vi "InitSensors.vi"   [LabVIEW 2019]
uses:
  <vilib>/Rock Robotics/SystemInterfaces/AI/FPGA_AIChannel.ctl
  <vilib>/Rock Robotics/WPI/ThirdParty/Phoenix-LabVIEW/Pigeon IMU/CTRE_PigeonIMU_TareType.ctl
  <vilib>/Rock Robotics/SystemInterfaces/DIO/FPGA_DIOChannel.ctl
  refnums.vi
  <vilib>/Rock Robotics/WPI/Counter/WPI_CounterDigitalInputToDigitalSource.vi
  <vilib>/Rock Robotics/WPI/Counter/WPI_CounterOpen UpDown Mode.vi
  <vilib>/Rock Robotics/WPI/Switch/WPI_SwitchOpenLimit.vi
  <vilib>/Rock Robotics/WPI/ThirdParty/Phoenix-LabVIEW/Pigeon IMU/CTRE_PigeonIMU_Open_TalonSRX.vi
types:
  T1 = typedef "FPGA_DIOChannel.ctl" = enum8{"DIO 0", "DIO 1", "DIO 2", "DIO 3", "DIO 4", "DIO 5", "DIO 6", "DIO 7", "DIO 8", "DIO 9", "DIO MXP 0", "DIO MXP 1", "DIO MXP 2", "DIO MXP 3", "DIO MXP 4", "DIO MXP 5", "DIO MXP 6", "DIO MXP 7", "DIO MXP 8", "DIO MXP 9", "DIO MXP 10", "DIO MXP 11", "DIO MXP 12", "DIO MXP 13", "DIO MXP 14", "DIO MXP 15", "SPI Port CS1", "SPI Port CS2", "SPI Port CS3", "SPI Port MISO", "SPI Port MOSI", "Invalid"}
  T2 = enum16{"Rising Edge", "Falling Edge", "Raising & Falling Edge", "Disabled"}
  T3 = typedef "FPGA_AIChannel.ctl" = enum8{"AI 0", "AI 1", "AI 2", "AI 3", "AI MXP 0", "AI MXP 1", "AI MXP 2", "AI MXP 3", "Invalid"}
  T4 = typedef "CTRE_PigeonIMU_TareType.ctl" = u8
  T5 = typedef "WPI_MotorControlDeviceRef.ctl" = cluster{"DeviceStatus":errorcluster, "Type":T6, "PWM":cluster{"PWM Channel":T7, "DeadBand":T8}, "CAN":cluster{"Device Number":u8, "SetOutput VI Ref":variant, "GetOutput VI Ref":variant, "Enable VI Ref":variant, "Disable VI Ref":variant, "Data":variant}, "Invert":bool, "DIO PWM":cluster{"PWM \"Enable\" Channel":T7, "DIOChannel":T1, "PWM Rate":dbl}}
  T6 = typedef "WPI_MotorControlType.ctl" = enum16{"PWM", "CAN", "DIO PWM"}
  T7 = typedef "FPGA_DIOPWMChannel.ctl" = enum8{"PWM 0", "PWM 1", "PWM 2", "PWM 3", "PWM 4", "PWM 5", "PWM 6", "PWM 7", "PWM 8", "PWM 9", "PWM MXP 0", "PWM MXP 1", "PWM MXP 2", "PWM MXP 3", "PWM MXP 4", "PWM MXP 5", "PWM MXP 6", "PWM MXP 7", "PWM MXP 8", "PWM MXP 9", "Invalid"}
  T8 = typedef "WPI_PWMDeadband.ctl" = cluster{"Name":string, "maxPositivePwm":i32, "minPositivePwm":i32, "centerPwm":i32, "maxNegativePwm":i32, "minNegativePwm":i32, "angularRange":u16}
  T9 = typedef "WPI_DigitalInputDevRef.ctl" = cluster{"DevStatus":errorcluster, "DIO Channel":T1}
  T10 = typedef "FPGA_CounterEncoderSourceConvertionLVSourceType.ctl" = cluster{"DevStatus":errorcluster, "AnalogTriggerMode?":bool, "DigitalMode":cluster{"DIO Channel":T11}, "AnalogTriggerMode":cluster{"AnalogTriggerIndex":T12, "OutputType":T13}}
  T11 = typedef "FPGA_DIODigitalSourceChannel.ctl" = enum8{"DIO 0", "DIO 1", "DIO 2", "DIO 3", "DIO 4", "DIO 5", "DIO 6", "DIO 7", "DIO 8", "DIO 9", "DIO MXP 0", "DIO MXP 1", "DIO MXP 2", "DIO MXP 3", "DIO MXP 4", "DIO MXP 5", "DIO MXP 6", "DIO MXP 7", "DIO MXP 8", "DIO MXP 9", "DIO MXP 10", "DIO MXP 11", "DIO MXP 12", "DIO MXP 13", "DIO MXP 14", "DIO MXP 15", "SPI Port CS1", "SPI Port CS2", "SPI Port CS3", "SPI Port MISO", "SPI Port MOSI", "Disabled"}
  T12 = typedef "FPGA_AnalogTriggerIndex.ctl" = enum8{"Trig 0", "Trig 1", "Trig 2", "Trig 3", "Trig 4", "Trig 5", "Trig 6", "Trig 7", "Invalid"}
  T13 = typedef "FPGA_AnalogTriggerOutType.ctl" = enum16{"InWindow", "TriggerState", "Rising", "Falling"}
  T14 = typedef "WPI_SwitchDevRef.ctl" = cluster{"DevStatus":errorcluster, "DIO Channel":T1, "CntIndex":T15, "Normally Closed":bool}
  T15 = typedef "FPGA_CounterCtrSystemIndex.ctl" = enum8{"Ctr 0", "Ctr 1", "Ctr 2", "Ctr 3", "Ctr 4", "Ctr 5", "Ctr 6", "Ctr 7", "Invalid"}
  T16 = typedef "WPI_PotentiometerDevRef.ctl" = cluster{"DevStatus":errorcluster, "Analog Channel":T3, "Invert Output":bool}
  T17 = typedef "CTRE_PigeonIMU_DeviceRef.ctl" = cluster{"DeviceStatus":errorcluster, "Device Number":u8, "Type":T18, "Device ID":u32, "Handle":u64, "UsageFrame":u32, "Library Path":path}
  T18 = typedef "CTRE_PigeonIMU_ConnectionType.ctl" = u32
  T19 = typedef "WPI_CounterDevRef.ctl" = cluster{"DevStatus":errorcluster, "CntIndex":T15}
  T20 = typedef "WPI_AnalogChannelDevRef.ctl" = cluster{"DevStatus":errorcluster, "Analog Channel":T3}
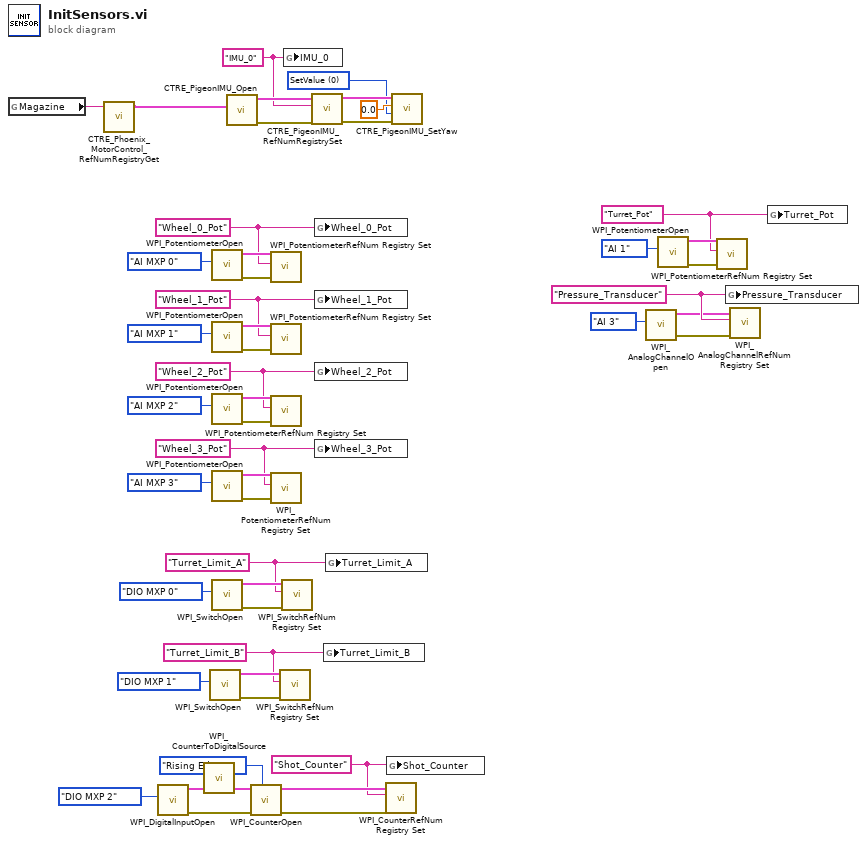
[diagram p0: block diagram]
diagram:
  w1 = "Turret_Limit_B"
  w5 = "Turret_Limit_A"
  w9 = "Shot_Counter"
  w18 = "Turret_Pot"
  w23 = T4 0 items=["SetValue"=0, "AddOffset"=1, "MatchCompass"=2, "SetOffset"=255] ("TareType (SetValue)")
  w27 = "IMU_0" ("refnum name")
  w32 = "Pressure_Transducer" ("Pressure_Transducer")
  w38 = "Wheel_3_Pot"
  w41 = "Wheel_2_Pot"
  w44 = "Wheel_1_Pot"
  w47 = "Wheel_0_Pot"
  n1 = global read "refnums.vi" "Magazine"() -> (w21:string)
  n2 = call <vilib>:"CTRE_Phoenix_MotorControl_RefNumRegistryGet.vi"("refnum name"=w21) -> ("PhoenixMotorControlDevRef"=w22:T5)  [unwired: 9 in, 1 out]
  n3 = call <vilib>:"WPI_DigitalInputOpen.vi"("DIO Channel"=FPGA_DIOChannel."DIO MXP 2" ("Source")) -> ("error out"=w12:errorcluster, "DigitalInputDevRef"=w14:T9)  [unwired: 1 in, 8 out]
  n4 = call-poly <vilib>:"WPI_CounterToDigitalSource.vi"("DigitalInputDevRef"=w14) -> ("Digital Source"=w16:T10)  [unwired: 6 out]
  n5 = call-poly <vilib>:"WPI_SwitchOpen.vi"("DIO Channel"=FPGA_DIOChannel."DIO MXP 1") -> ("error out"=w3:errorcluster, "SwitchDevRef"=w4:T14)  [unwired: 9 in]
  n6 = call <vilib>:"WPI_PotentiometerOpen.vi"("Analog Channel"=FPGA_AIChannel."AI MXP 0") -> ("error out"=w37:errorcluster, "PotDevRef"=w49:T16)  [unwired: 9 in]
  n7 = call <vilib>:"WPI_PotentiometerOpen.vi"("Analog Channel"=FPGA_AIChannel."AI MXP 1") -> ("error out"=w36:errorcluster, "PotDevRef"=w46:T16)  [unwired: 9 in]
  n8 = call <vilib>:"WPI_PotentiometerOpen.vi"("Analog Channel"=FPGA_AIChannel."AI MXP 2") -> ("error out"=w35:errorcluster, "PotDevRef"=w43:T16)  [unwired: 9 in]
  n9 = call <vilib>:"WPI_PotentiometerOpen.vi"("Analog Channel"=FPGA_AIChannel."AI MXP 3") -> ("error out"=w34:errorcluster, "PotDevRef"=w40:T16)  [unwired: 9 in]
  n10 = call-poly <vilib>:"WPI_SwitchOpen.vi"("DIO Channel"=FPGA_DIOChannel."DIO MXP 0") -> ("error out"=w7:errorcluster, "SwitchDevRef"=w8:T14)  [unwired: 9 in]
  n11 = call-poly <vilib>:"CTRE_PigeonIMU_Open.vi"("CAN Talon SRX Ref"=w22) -> ("error out"=w28:errorcluster, "PigeonIMUDevRef"=w29:T17)  [unwired: 9 in]
  n12 = call-poly <vilib>:"WPI_CounterOpen.vi"("UpEdge"=T2."Rising Edge", "error in (no error)"=w12, "Up Source"=w16) -> ("error out"=w11:errorcluster, "CounterDevRef"=w10:T19)  [unwired: 4 in, 3 out]
  n13 = call <vilib>:"WPI_PotentiometerRefNum Registry Set.vi"("error in (no error)"=w37, "refnum name"=w47, "PotDevRef"=w49) -> ()  [unwired: 7 in, 2 out]
  n14 = call <vilib>:"WPI_PotentiometerRefNum Registry Set.vi"("error in (no error)"=w36, "refnum name"=w44, "PotDevRef"=w46) -> ()  [unwired: 7 in, 2 out]
  n15 = call <vilib>:"WPI_PotentiometerRefNum Registry Set.vi"("error in (no error)"=w35, "refnum name"=w41, "PotDevRef"=w43) -> ()  [unwired: 7 in, 2 out]
  n16 = call <vilib>:"WPI_PotentiometerRefNum Registry Set.vi"("error in (no error)"=w34, "refnum name"=w38, "PotDevRef"=w40) -> ()  [unwired: 7 in, 2 out]
  n17 = call <vilib>:"WPI_SwitchRefNum Registry Set.vi"("error in (no error)"=w3, "refnum name"=w1, "SwitchDevRef"=w4) -> ()  [unwired: 7 in, 2 out]
  n18 = call <vilib>:"WPI_SwitchRefNum Registry Set.vi"("error in (no error)"=w7, "refnum name"=w5, "SwitchDevRef"=w8) -> ()  [unwired: 7 in, 2 out]
  n19 = global write "refnums.vi" "IMU_0"(w27) -> ()
  n20 = call <vilib>:"CTRE_PigeonIMU_RefNumRegistrySet.vi"("error in (no error)"=w28, "refnum name"=w27, "PigeonIMUDevRef"=w29) -> ("error out"=w25:errorcluster, "PigeonIMUDevRef"=w26:T17)  [unwired: 7 in]
  n21 = global write "refnums.vi" "Wheel_0_Pot"(w47) -> ()
  n22 = global write "refnums.vi" "Wheel_1_Pot"(w44) -> ()
  n23 = global write "refnums.vi" "Wheel_2_Pot"(w41) -> ()
  n24 = global write "refnums.vi" "Wheel_3_Pot"(w38) -> ()
  n25 = global write "refnums.vi" "Turret_Limit_B"(w1) -> ()
  n26 = global write "refnums.vi" "Turret_Limit_A"(w5) -> ()
  n27 = call <vilib>:"WPI_CounterRefNum Registry Set.vi"("error in (no error)"=w11, "refnum name"=w9, "CounterDevRef"=w10) -> ()  [unwired: 7 in, 2 out]
  n28 = global write "refnums.vi" "Shot_Counter"(w9) -> ()
  n29 = call <vilib>:"CTRE_PigeonIMU_SetYaw.vi"("error in (no error)"=w25, "TareType (SetValue)"=w23, "Value"=0.0, "PigeonIMUDevRef"=w26) -> ()  [unwired: 6 in, 2 out]
  n30 = call <vilib>:"WPI_AnalogChannelOpen.vi"("Analog Channel"=FPGA_AIChannel."AI 3") -> ("error out"=w30:errorcluster, "AIDeviceRef"=w31:T20)  [unwired: 9 in]
  n31 = call <vilib>:"WPI_PotentiometerOpen.vi"("Analog Channel"=FPGA_AIChannel."AI 1") -> ("error out"=w17:errorcluster, "PotDevRef"=w20:T16)  [unwired: 9 in]
  n32 = call <vilib>:"WPI_PotentiometerRefNum Registry Set.vi"("error in (no error)"=w17, "refnum name"=w18, "PotDevRef"=w20) -> ()  [unwired: 7 in, 2 out]
  n33 = global write "refnums.vi" "Pressure_Transducer"(w32) -> ()
  n34 = call <vilib>:"WPI_AnalogChannelRefNum Registry Set.vi"("error in (no error)"=w30, "refnum name"=w32, "AIDeviceRef"=w31) -> ()  [unwired: 7 in, 2 out]
  n35 = global write "refnums.vi" "Turret_Pot"(w18) -> ()
